vi "DETH_GPIT_COMBI_VR_COM5_COM7_hex_VE_FP_STOP_VE_BR_NEW.vi"() -> ()   [LabVIEW 2009]
uses:
  <vilib>/Instr/_visa.llb/VISA Configure Serial Port (Instr).vi
panel:
  in  "GPIT Backlash":i32
  in  "DETT Backlash":i32
  in  "DETH/GPIT":dbl max=1.0 step=1.0
  out "GPIT Status":string
  out "read buffer 3":string
  out "GPIT":i32
  out "GPIT Range?":bool
  out "GPIT rev/sec":dbl caption="Velocity"
  out "GPIT MINPOS":i32=-94296
  out "GPIT MAXPOS":i32=-34296
  out "GPIT COM PORT":refnum<visa-resource-name>="COM5"
  out "GPIT Step":i32
  in  "Stop":bool
  out "DETH Range?":bool
  out "DETH":i32
  out "read buffer 2":string
  out "DETH Status":string
  out "DETH rev//sec":dbl caption="Velocity"
  in  "Go":bool
  in  "DETH Step":i32=-1000 min=-1000 max=1000 step=100
  out "DETH MINPOS":i32=-94296
  out "DETH MAXPOS":i32=-34296
  out "DETT COM PORT":refnum<visa-resource-name>="COM5"
  # "DETH COM5 & GPIT COM7"
  # "20000 steps/rev\n2.5mm/rev\n0.05rev/sec"
  # "20000 steps/rev\n1 mm/rev\n0.01rev/sec"
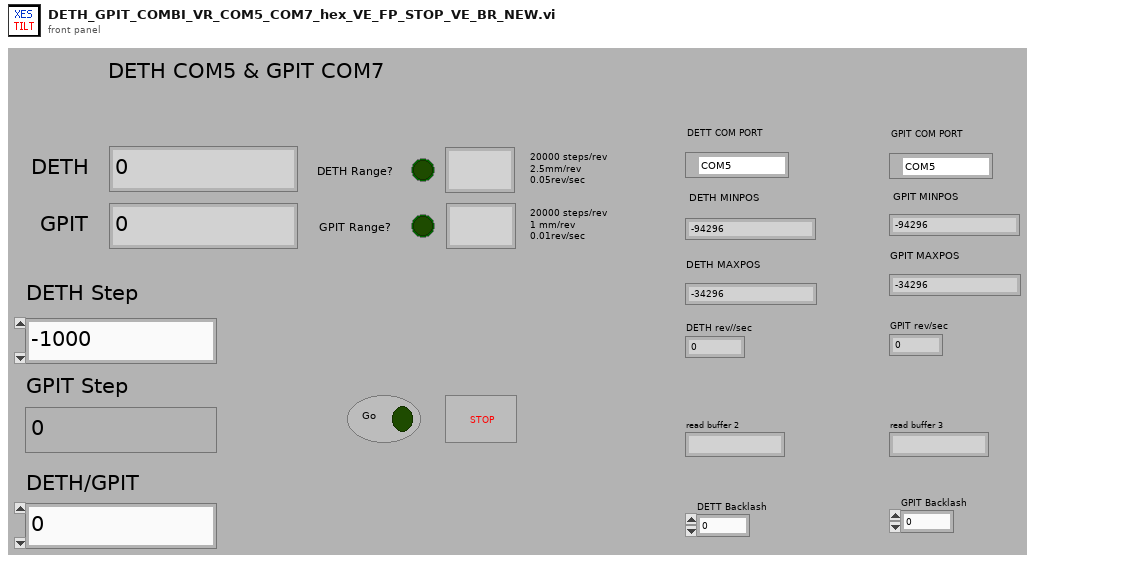
[diagram p1: front panel]
types:
  T1 = enum16{"Power-up Signature", "Accel Rate", "Accel Max", "Bit Rate", "Buffer Status", "Change Current", "Commence Jogging", "Change Jog Speed", "Continue", "Define Address", "Distance for FC,FM,FO,FY", "Decel Rate", "Distance or Position", "Define Limits", "Encoder Deadband", "Encoder Function", "Encoder Position", "Encoder Ratio", "Feed to Length with Speed Change", "Feed to Length", "Feed to Sensor with Mask Dist", "Feed to Length & Set Output", "Feed to Position", "Feed to Sensor", "Feed to Sensor w/safety", "Follow Handwheel", "Immediate Distance?", "Immediate Encoder?", "Immediate Low Output", "Immediate High Output", "Immediate Position?", "Input Status?", "Jog Accel/Decel", "Jog Disable", "Jog Enable", "Jog Speed", "Motor Disable", "Motor Enable", "Microstep Resolution", "Power up Current", "Power up Mode", "Pause", "Request Status", "Revision Level?", "Seek Home", "Stop Jogging", "Stop & Kill Buffer", "Set Output", "Set ABS Position", "Send String", "Stop", "Velocity for Speed Change", "Velocity Setting", "Wait for Input", "Wait Time"}
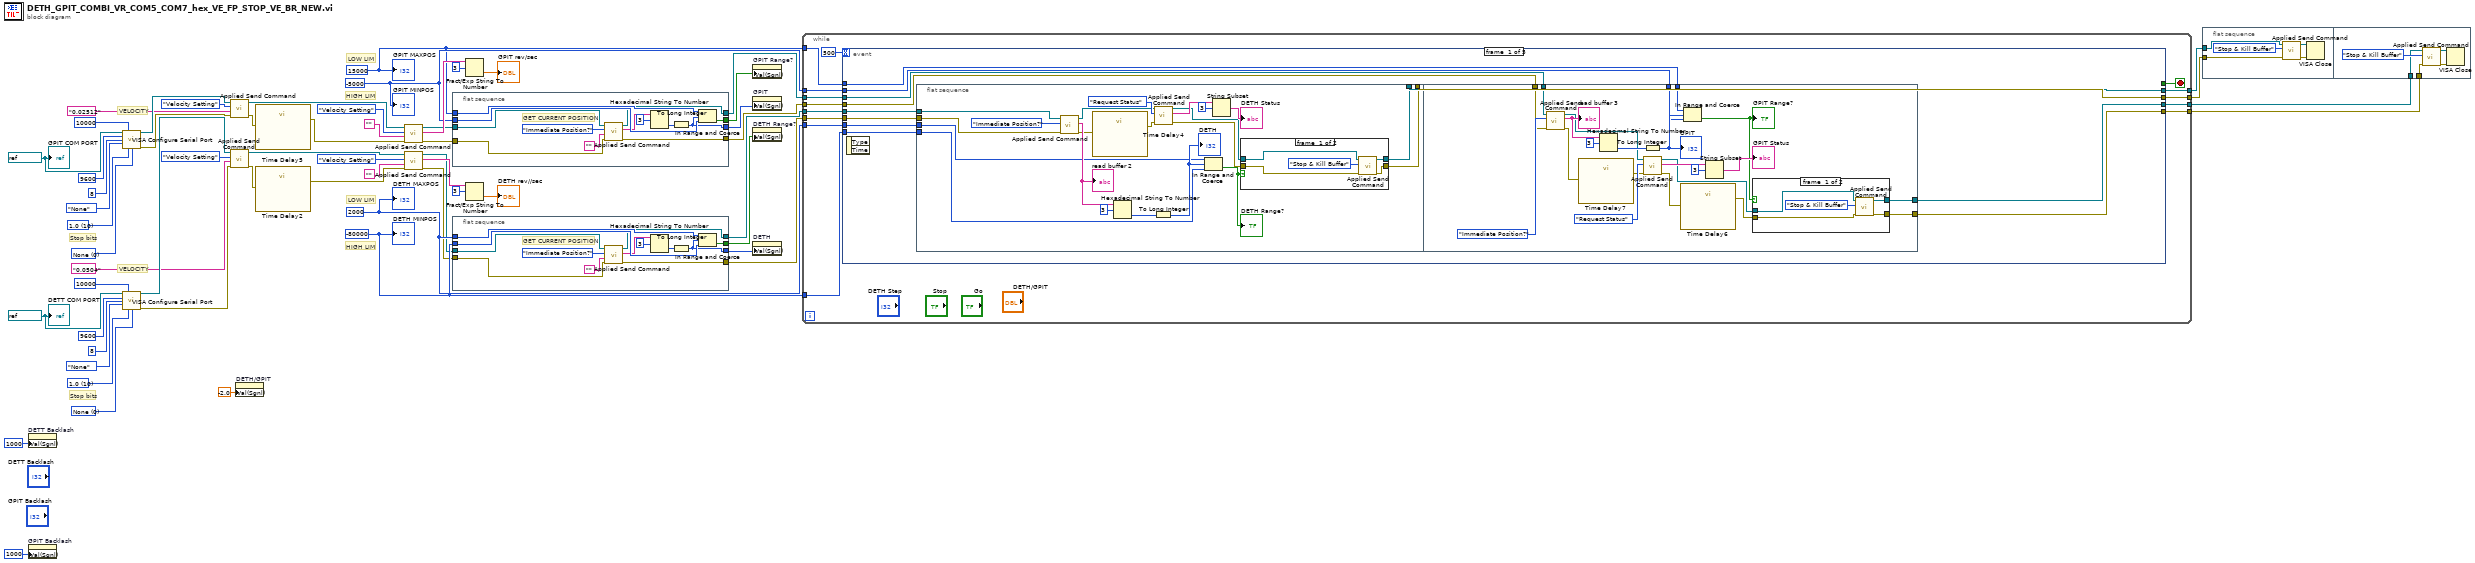
[diagram p0: block diagram]
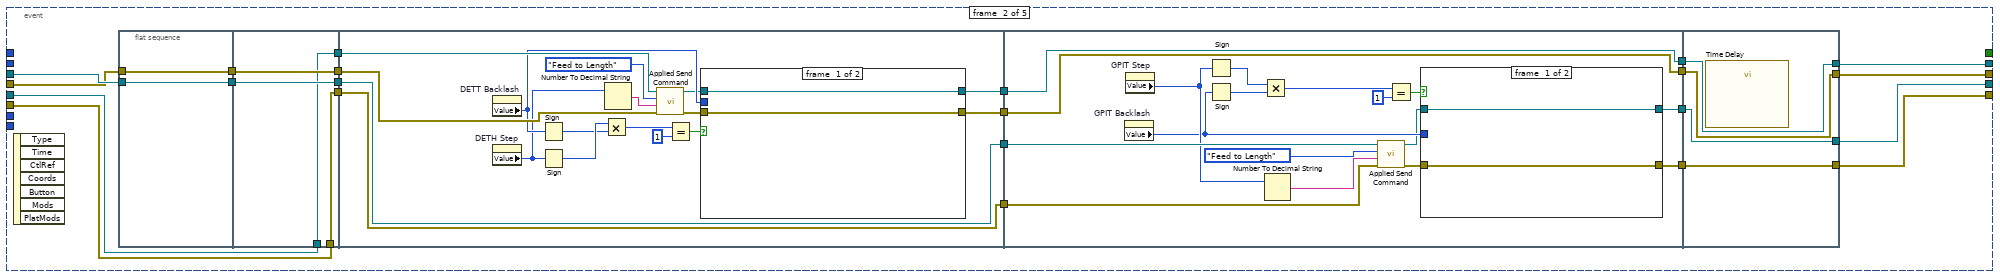
[diagram p4: hidden frame]
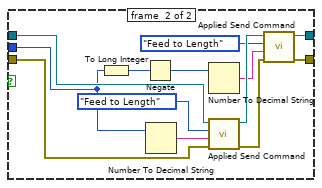
[diagram p5: hidden frame]
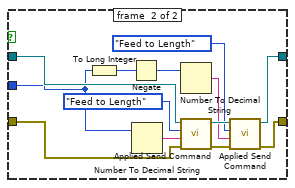
[diagram p6: hidden frame]
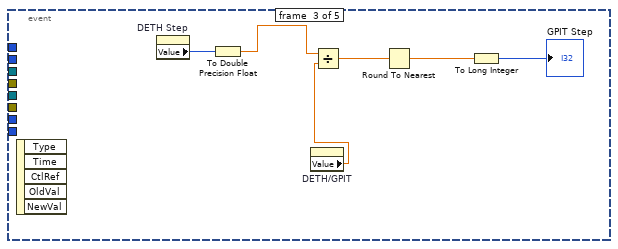
[diagram p7: hidden frame]
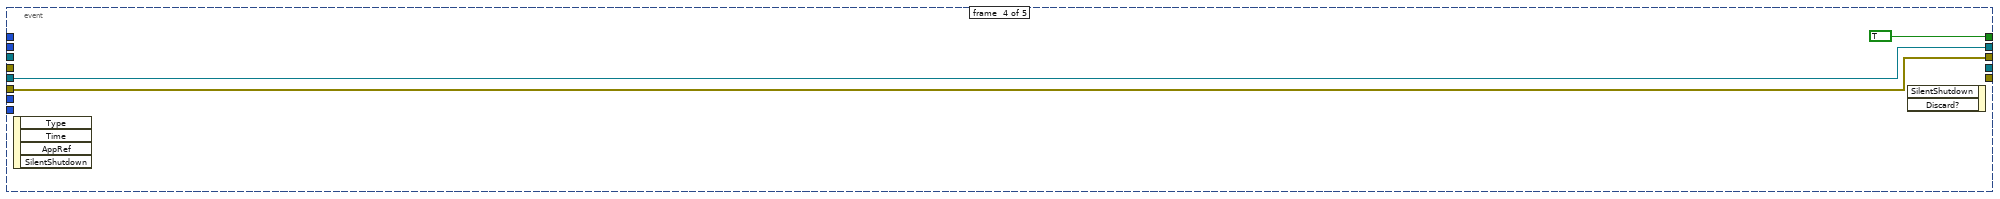
[diagram p8: hidden frame]
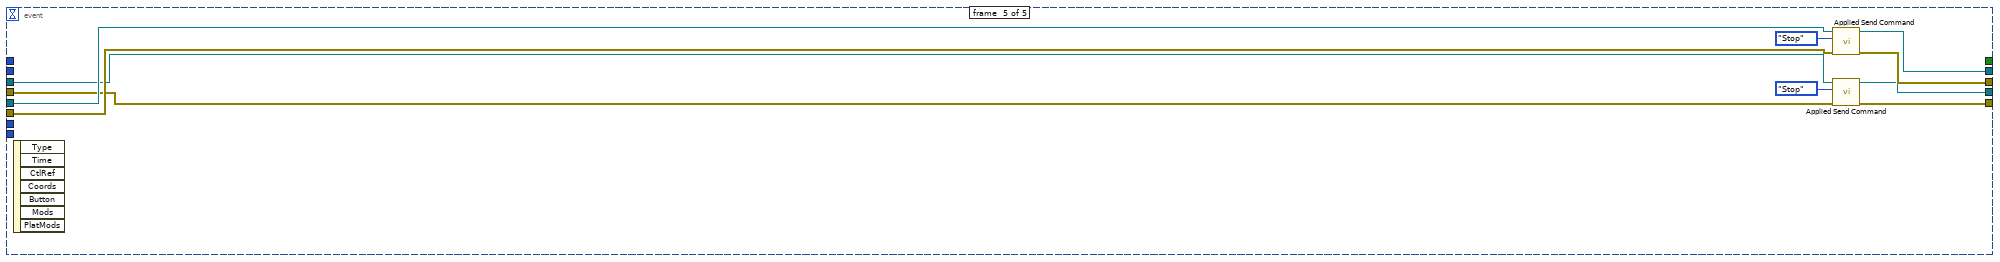
[diagram p9: hidden frame]
diagram:
  w12 = -5000 ("lower limit")
  w11 = 15000 ("upper limit")
  w27 = refnum<visa-resource-name> "COM7" ("COM PORT")
  w29 = u16 0 items=["None", "XON/XOFF", "RTS/CTS", "XON/XOFF & RTS/CTS", "DTR/DSR", "XON/XOFF & DTR/DSR"] ("flow control (0:none)")
  w30 = u16 10 items=["1.0"=10, "1.5"=15, "2.0"=20] ("stop bits (10: 1 bit)")
  w51 = -80000 ("lower limit")
  w52 = 2000 ("upper limit")
  w55 = refnum<visa-resource-name> "COM5" ("COM PORT")
  w57 = u16 0 items=["None", "XON/XOFF", "RTS/CTS", "XON/XOFF & RTS/CTS", "DTR/DSR", "XON/XOFF & DTR/DSR"] ("flow control (0:none)")
  w58 = u16 10 items=["1.0"=10, "1.5"=15, "2.0"=20] ("stop bits (10: 1 bit)")
  # "VELOCITY"
  # "HIGH LIM"
  # "LOW LIM"
  # "Stop bits"
  # "VELOCITY"
  # "HIGH LIM"
  # "LOW LIM"
  # "Stop bits"
  n1 = property on="DETT Backlash" class="DigNum (strict)"("Val(Sgnl)"=1000 ("Value (Signaling)")) -> ()  [unwired: 2 in, 2 out]
  n2 = property on="GPIT Backlash" class="DigNum (strict)"("Val(Sgnl)"=1000 ("Value (Signaling)")) -> ()  [unwired: 2 in, 2 out]
  n3 = call-poly "VISA Configure Serial Port"("VISA resource name"=w27, "timeout (10sec)"=u32 10000, "baud rate (9600)"=u32 9600, "data bits (8)"=u16 8, "parity (0:none)"=enum16{"None", "Odd", "Even", "Mark", "Space"}."None", "stop bits (10: 1 bit)"=w30, "flow control (0:none)"=w29) -> ("VISA resource name out"=w15:refnum<visa-resource-name>, "error out"=w14:errorcluster)  [unwired: 7 in]
  n4 = call-poly "VISA Configure Serial Port"("VISA resource name"=w55, "timeout (10sec)"=u32 10000, "baud rate (9600)"=u32 9600, "data bits (8)"=u16 8, "parity (0:none)"=enum16{"None", "Odd", "Even", "Mark", "Space"}."None", "stop bits (10: 1 bit)"=w58, "flow control (0:none)"=w57) -> ("VISA resource name out"=w37:refnum<visa-resource-name>, "error out"=w36:errorcluster)  [unwired: 7 in]
  n5 = call "Applied Send Command.vi"("error in (no error)"=w14, "Extra"="0.02512", "Command"=T1."Velocity Setting", "VISA resource name"=w15) -> ("error out"=w25:errorcluster, "VISA resource name out"=w20:refnum<visa-resource-name>)  [unwired: 3 in, 1 out]
  n6 = call "Applied Send Command.vi"("error in (no error)"=w36, "Extra"="0.0504", "Command"=T1."Velocity Setting", "VISA resource name"=w37) -> ("error out"=w49:errorcluster, "VISA resource name out"=w44:refnum<visa-resource-name>)  [unwired: 3 in, 1 out]
  n7 = property on="DETH/GPIT" class="DigNum (strict)"("Val(Sgnl)"=-2.0 ("Value (Signaling)")) -> ()  [unwired: 2 in, 2 out]
  n8 = call "Time Delay5"("error in (no error)"=w25) -> ("error out"=w21:errorcluster)  [unwired: 10 in]
  n9 = call "Time Delay2"("error in (no error)"=w49) -> ("error out"=w45:errorcluster)  [unwired: 10 in]
  n10 = call "Applied Send Command.vi"("error in (no error)"=w21, "Extra"="", "Command"=T1."Velocity Setting", "VISA resource name"=w20) -> ("error out"=w18:errorcluster, "read buffer"=w23:string, "VISA resource name out"=w19:refnum<visa-resource-name>)  [unwired: 3 in]
  n11 = call "Applied Send Command.vi"("error in (no error)"=w45, "Extra"="", "Command"=T1."Velocity Setting", "VISA resource name"=w44) -> ("error out"=w42:errorcluster, "read buffer"=w47:string, "VISA resource name out"=w43:refnum<visa-resource-name>)  [unwired: 3 in]
  n12 = flat-sequence {
    tunnel: w18 -> [w74]
    tunnel: w19 -> [w73]
    tunnel: w11 -> [w71]
    tunnel: w12 -> [w70]
    tunnel: [w72] -> w9
    tunnel: [w62] -> w4
    tunnel: [w69] -> w6
    tunnel: [w68] -> w10
    frame #0 {
      # "GET CURRENT POSITION"
      n13 = call "Applied Send Command.vi"("error in (no error)"=w74, "Extra"="", "Command"=T1."Immediate Position?", "VISA resource name"=w73) -> ("error out"=w72:errorcluster, "read buffer"=w66:string, "VISA resource name out"=w68:refnum<visa-resource-name>)  [unwired: 3 in]
      n14 = Hexadecimal String To Number(string=w66, offset=3) -> (number=w63:u32)  [unwired: 1 in, 1 out]
      n15 = To Long Integer(number=w63) -> (32bit integer=w62:i32)
      n16 = In Range and Coerce(upper limit=w71, x=w62, lower limit=w70) -> (In Range?=w69:bool)  [unwired: 1 out]
    }
  }
  n17 = flat-sequence {
    tunnel: w42 -> [w87]
    tunnel: w43 -> [w86]
    tunnel: w52 -> [w85]
    tunnel: w51 -> [w84]
    tunnel: [w75] -> w53
    tunnel: [w76] -> w5
    tunnel: [w83] -> w34
    tunnel: [w82] -> w54
    frame #0 {
      # "GET CURRENT POSITION"
      n18 = call "Applied Send Command.vi"("error in (no error)"=w87, "Extra"="", "Command"=T1."Immediate Position?", "VISA resource name"=w86) -> ("error out"=w75:errorcluster, "read buffer"=w80:string, "VISA resource name out"=w82:refnum<visa-resource-name>)  [unwired: 3 in]
      n19 = Hexadecimal String To Number(string=w80, offset=3) -> (number=w77:u32)  [unwired: 1 in, 1 out]
      n20 = To Long Integer(number=w77) -> (32bit integer=w76:i32)
      n21 = In Range and Coerce(upper limit=w85, x=w76, lower limit=w84) -> (In Range?=w83:bool)  [unwired: 1 out]
    }
  }
  n22 = Fract/Exp String To Number(string=w23, offset=3) -> (number=→"GPIT rev/sec":dbl)  [unwired: 2 in, 1 out]
  n23 = Fract/Exp String To Number(string=w47, offset=3) -> (number=→"DETH rev//sec":dbl)  [unwired: 2 in, 1 out]
  n24 = property on="GPIT Range?" class="Bool (strict)"("Val(Sgnl)"=w6) -> ()  [unwired: 2 in, 2 out]
  n25 = property on="GPIT" class="DigNum (strict)"("Val(Sgnl)"=w4) -> ()  [unwired: 2 in, 2 out]
  n26 = property on="DETH Range?" class="Bool (strict)"("Val(Sgnl)"=w34) -> ()  [unwired: 2 in, 2 out]
  n27 = property on="DETH" class="DigNum (strict)"("Val(Sgnl)"=w5) -> ()  [unwired: 2 in, 2 out]
  n28 = while {
    tunnel: w54 -> [w95]
    tunnel: w53 -> [w100]
    tunnel: [w101] -> w38
    tunnel: [w99] -> w39
    tunnel: w52 -> [w98]
    tunnel: w51 -> [w97]
    tunnel: w12 -> [w93]
    tunnel: w11 -> [w88]
    tunnel: w10 -> [w92]
    tunnel: w9 -> [w91]
    tunnel: [w90] -> w8
    tunnel: [w89] -> w7
    stop <- w94 stop-if-true
    n29 = event shown="[1] \"Go\": Mouse Up" {
      selector: _ -> [_ _ _ _ _]
      dyn-events: _ -> [_ _ _ _ _]
      timeout: 500 -> [_ _ _ _ _]
      tunnel: w100 -> [w111 w172 _ w274 w283]
      tunnel: [w105 w179 _ w274 w281] -> w101
      tunnel: w95 -> [w110 w171 _ w275 w284]
      tunnel: [w104 w192 _ w275 w282] -> w99
      tunnel: w98 -> [w113 _ _ _ _]
      tunnel: w97 -> [w112 _ _ _ _]
      tunnel: [_ _ _ TRUE _] -> w94
      tunnel: w93 -> [w102 _ _ _ _]
      tunnel: w88 -> [w103 _ _ _ _]
      tunnel: w92 -> [w109 w187 _ _ w277]
      tunnel: w91 -> [w108 w183 _ _ w276]
      tunnel: [w107 w177 _ _ w279] -> w90
      tunnel: [w106 w175 _ _ w278] -> w89
      event #0 {
        n30 = event-data() -> ()  [unwired: 1 in, 2 out]
        n31 = flat-sequence {
          tunnel: w112 -> [w134]
          tunnel: w113 -> [w126]
          tunnel: w111 -> [w125]
          tunnel: w110 -> [w124]
          tunnel: [w116] -> w104
          tunnel: [w114] -> w105
          tunnel: w109 -> [w150]
          tunnel: w108 -> [w149]
          tunnel: w103 -> [w148]
          tunnel: w102 -> [w147]
          tunnel: [w144] -> w107
          tunnel: [w145] -> w106
          frame #0 {
            n32 = call "Applied Send Command.vi"("error in (no error)"=w125, "Command"=T1."Immediate Position?", "VISA resource name"=w124) -> ("error out"=w120:errorcluster, "read buffer"=w132:string, "VISA resource name out"=w127:refnum<visa-resource-name>)  [unwired: 4 in]
            "read buffer 2" <- w132
            n33 = call "Time Delay4"("error in (no error)"=w120) -> ("error out"=w119:errorcluster)  [unwired: 10 in]
            n34 = Hexadecimal String To Number(string=w132, offset=3) -> (number=w131:u32)  [unwired: 1 in, 1 out]
            n35 = call "Applied Send Command.vi"("error in (no error)"=w119, "Command"=T1."Request Status", "VISA resource name"=w127) -> ("error out"=w115:errorcluster, "read buffer"=w123:string, "VISA resource name out"=w117:refnum<visa-resource-name>)  [unwired: 4 in]
            n36 = To Long Integer(number=w131) -> (32bit integer=w129:i32)
            "DETH" <- w129
            n37 = In Range and Coerce(upper limit=w126, x=w129, lower limit=w134) -> (In Range?=w118:bool)  [unwired: 1 out]
            "DETH Range?" <- w118
            n38 = String Subset(string=w123, offset (0)=3) -> (substring=→"DETH Status":string)  [unwired: 1 in]
            n39 = case shown="False" w118 {
              tunnel: w117 -> [w136 w141]
              tunnel: [w138 w141] -> w116
              tunnel: [w139 w140] -> w114
              tunnel: w115 -> [w135 w140]
              frame #0 {
                n40 = call "Applied Send Command.vi"("error in (no error)"=w135, "Command"=T1."Stop & Kill Buffer", "VISA resource name"=w136) -> ("error out"=w139:errorcluster, "VISA resource name out"=w138:refnum<visa-resource-name>)  [unwired: 4 in, 1 out]
              }
              frame #1 {
              }
            }
          }
          frame #1 {
            n41 = call "Applied Send Command.vi"("error in (no error)"=w149, "Command"=T1."Immediate Position?", "VISA resource name"=w150) -> ("error out"=w152:errorcluster, "read buffer"=w162:string, "VISA resource name out"=w157:refnum<visa-resource-name>)  [unwired: 4 in]
            "read buffer 3" <- w162
            n42 = call "Time Delay7"("error in (no error)"=w152) -> ("error out"=w151:errorcluster)  [unwired: 10 in]
            n43 = Hexadecimal String To Number(string=w162, offset=3) -> (number=w161:u32)  [unwired: 1 in, 1 out]
            n44 = To Long Integer(number=w161) -> (32bit integer=w159:i32)
            "GPIT" <- w159
            n45 = call "Applied Send Command.vi"("error in (no error)"=w151, "Command"=T1."Request Status", "VISA resource name"=w157) -> ("error out"=w156:errorcluster, "read buffer"=w155:string, "VISA resource name out"=w143:refnum<visa-resource-name>)  [unwired: 4 in]
            n46 = call "Time Delay6"("error in (no error)"=w156) -> ("error out"=w146:errorcluster)  [unwired: 10 in]
            n47 = In Range and Coerce(upper limit=w148, x=w159, lower limit=w147) -> (In Range?=w142:bool)  [unwired: 1 out]
            "GPIT Range?" <- w142
            n48 = String Subset(string=w155, offset (0)=3) -> (substring=→"GPIT Status":string)  [unwired: 1 in]
            n49 = case shown="False" w142 {
              tunnel: w143 -> [w165 w170]
              tunnel: [w167 w170] -> w144
              tunnel: [w168 w169] -> w145
              tunnel: w146 -> [w164 w169]
              frame #0 {
                n50 = call "Applied Send Command.vi"("error in (no error)"=w164, "Command"=T1."Stop & Kill Buffer", "VISA resource name"=w165) -> ("error out"=w168:errorcluster, "VISA resource name out"=w167:refnum<visa-resource-name>)  [unwired: 4 in, 1 out]
              }
              frame #1 {
              }
            }
          }
        }
      }
      event #1 {
        n51 = event-data() -> ()  [unwired: 1 in, 7 out]
        n52 = flat-sequence {
          tunnel: w187 -> [w194]
          tunnel: [w194] -> w186
          tunnel: [w193] -> w184
          tunnel: w183 -> [w193]
          tunnel: [w198] -> w189
          tunnel: w186 -> [w198]
          tunnel: [w197] -> w185
          tunnel: w184 -> [w197]
          tunnel: [w196] -> w174
          tunnel: [w195] -> w173
          tunnel: w172 -> [w195]
          tunnel: w171 -> [w196]
          tunnel: [w200] -> w191
          tunnel: w189 -> [w214]
          tunnel: [w214] -> w188
          tunnel: w185 -> [w212]
          tunnel: [w211] -> w182
          tunnel: [w199] -> w181
          tunnel: w174 -> [w213]
          tunnel: w173 -> [w211]
          tunnel: w191 -> [w247]
          tunnel: [w247] -> w190
          tunnel: w188 -> [w245]
          tunnel: w182 -> [w244]
          tunnel: w181 -> [w243]
          tunnel: [w243] -> w180
          tunnel: [w231] -> w178
          tunnel: [w233] -> w176
          tunnel: [w266] -> w192
          tunnel: w190 -> [w266]
          tunnel: w180 -> [w265]
          tunnel: [w265] -> w179
          tunnel: w178 -> [w264]
          tunnel: [w264] -> w177
          tunnel: [w263] -> w175
          tunnel: w176 -> [w263]
          frame #0 {
          }
          frame #1 {
          }
          frame #2 {
            n53 = property on="DETT Backlash" class="DigNum (strict)"() -> ("Value"=w204:i32)  [unwired: 2 in, 2 out]
            n54 = property on="DETH Step" class="DigNum (strict)"() -> ("Value"=w203:i32)  [unwired: 2 in, 2 out]
            n55 = Sign(1:w204) -> (0:w208:i32)
            n56 = Sign(1:w203) -> (0:w209:i32)
            n57 = Multiply(x=w209, y=w208) -> (x*y=w207:i32)
            n58 = Number To Decimal String(number=w203) -> (decimal integer string=w210:string)  [unwired: 1 in]
            n59 = call "Applied Send Command.vi"("error in (no error)"=w212, "Extra"=w210, "Command"=T1."Feed to Length", "VISA resource name"=w213) -> ("error out"=w201:errorcluster, "VISA resource name out"=w202:refnum<visa-resource-name>)  [unwired: 3 in, 1 out]
            n60 = Equal?(x=w207, y=1) -> (x = y?=w205:bool)
            n61 = case shown="True" w205 {
              tunnel: w202 -> [w217 w229]
              tunnel: [w217 w223] -> w200
              tunnel: [w216 w224] -> w199
              tunnel: w201 -> [w216 w228]
              tunnel: w204 -> [_ w218]
              frame #0 {
              }
              frame #1 {
                n62 = To Long Integer(number=w218) -> (32bit integer=w221:i32)
                n63 = Negate(x=w221) -> (-x=w222:i32)
                n64 = Number To Decimal String(number=w218) -> (decimal integer string=w227:string)  [unwired: 1 in]
                n65 = Number To Decimal String(number=w222) -> (decimal integer string=w220:string)  [unwired: 1 in]
                n66 = call "Applied Send Command.vi"("error in (no error)"=w228, "Extra"=w227, "Command"=T1."Feed to Length", "VISA resource name"=w229) -> ("error out"=w225:errorcluster, "VISA resource name out"=w226:refnum<visa-resource-name>)  [unwired: 3 in, 1 out]
                n67 = call "Applied Send Command.vi"("error in (no error)"=w225, "Extra"=w220, "Command"=T1."Feed to Length", "VISA resource name"=w226) -> ("error out"=w224:errorcluster, "VISA resource name out"=w223:refnum<visa-resource-name>)  [unwired: 3 in, 1 out]
              }
            }
          }
          frame #3 {
            n68 = property on="GPIT Backlash" class="DigNum (strict)"() -> ("Value"=w235:i32)  [unwired: 2 in, 2 out]
            n69 = property on="GPIT Step" class="DigNum (strict)"() -> ("Value"=w237:i32)  [unwired: 2 in, 2 out]
            n70 = Sign(1:w237) -> (0:w241:i32)
            n71 = Sign(1:w235) -> (0:w240:i32)
            n72 = Multiply(x=w241, y=w240) -> (x*y=w239:i32)
            n73 = Number To Decimal String(number=w237) -> (decimal integer string=w242:string)  [unwired: 1 in]
            n74 = call "Applied Send Command.vi"("error in (no error)"=w244, "Extra"=w242, "Command"=T1."Feed to Length", "VISA resource name"=w245) -> ("error out"=w234:errorcluster, "VISA resource name out"=w232:refnum<visa-resource-name>)  [unwired: 3 in, 1 out]
            n75 = Equal?(x=w239, y=1) -> (x = y?=w236:bool)
            n76 = case shown="True" w236 {
              tunnel: w232 -> [w249 w261]
              tunnel: [w249 w255] -> w231
              tunnel: [w248 w256] -> w233
              tunnel: w234 -> [w248 w260]
              tunnel: w235 -> [_ w250]
              frame #0 {
              }
              frame #1 {
                n77 = To Long Integer(number=w250) -> (32bit integer=w253:i32)
                n78 = Negate(x=w253) -> (-x=w254:i32)
                n79 = Number To Decimal String(number=w250) -> (decimal integer string=w259:string)  [unwired: 1 in]
                n80 = Number To Decimal String(number=w254) -> (decimal integer string=w252:string)  [unwired: 1 in]
                n81 = call "Applied Send Command.vi"("error in (no error)"=w260, "Extra"=w259, "Command"=T1."Feed to Length", "VISA resource name"=w261) -> ("error out"=w257:errorcluster, "VISA resource name out"=w258:refnum<visa-resource-name>)  [unwired: 3 in, 1 out]
                n82 = call "Applied Send Command.vi"("error in (no error)"=w257, "Extra"=w252, "Command"=T1."Feed to Length", "VISA resource name"=w258) -> ("error out"=w256:errorcluster, "VISA resource name out"=w255:refnum<visa-resource-name>)  [unwired: 3 in, 1 out]
              }
            }
          }
          frame #4 {
            n83 = call "Time Delay"() -> ()  [unwired: 11 in, 1 out]
          }
        }
      }
      event #2 {
        n84 = event-data() -> ()  [unwired: 1 in, 5 out]
        n85 = property on="DETH Step" class="DigNum (strict)"() -> ("Value"=w268:i32)  [unwired: 2 in, 2 out]
        n86 = To Double Precision Float(number=w268) -> (double precision float=w269:dbl)
        n87 = property on="DETH/GPIT" class="DigNum (strict)"() -> ("Value"=w267:dbl)  [unwired: 2 in, 2 out]
        n88 = Divide(x=w269, y=w267) -> (x/y=w272:dbl)
        n89 = Round To Nearest(number=w272) -> (nearest integer value=w271:dbl)
        n90 = To Long Integer(number=w271) -> (32bit integer=→"GPIT Step":i32)
      }
      event #3 {
        n91 = event-data() -> ()  [unwired: 1 in, 4 out]
        n92 = event-data() -> ()  [unwired: 3 in, 1 out]
      }
      event #4 {
        n93 = event-data() -> ()  [unwired: 1 in, 7 out]
        n94 = call "Applied Send Command.vi"("error in (no error)"=w283, "Command"=T1."Stop", "VISA resource name"=w284) -> ("error out"=w281:errorcluster, "VISA resource name out"=w282:refnum<visa-resource-name>)  [unwired: 4 in, 1 out]
        n95 = call "Applied Send Command.vi"("error in (no error)"=w276, "Command"=T1."Stop", "VISA resource name"=w277) -> ("error out"=w278:errorcluster, "VISA resource name out"=w279:refnum<visa-resource-name>)  [unwired: 4 in, 1 out]
      }
    }
  }
  n96 = flat-sequence {
    tunnel: w39 -> [w289]
    tunnel: w38 -> [w286]
    tunnel: w8 -> [w291]
    tunnel: w7 -> [w292]
    frame #0 {
      n97 = call "Applied Send Command.vi"("error in (no error)"=w286, "Command"=T1."Stop & Kill Buffer", "VISA resource name"=w289) -> ("error out"=w287:errorcluster, "VISA resource name out"=w288:refnum<visa-resource-name>)  [unwired: 4 in, 1 out]
      n98 = VISA Close(VISA resource name=w288, error in (no error)=w287) -> ()  [unwired: 1 out]
    }
    frame #1 {
      n99 = call "Applied Send Command.vi"("error in (no error)"=w292, "Command"=T1."Stop & Kill Buffer", "VISA resource name"=w291) -> ("error out"=w293:errorcluster, "VISA resource name out"=w294:refnum<visa-resource-name>)  [unwired: 4 in, 1 out]
      n100 = VISA Close(VISA resource name=w294, error in (no error)=w293) -> ()  [unwired: 1 out]
    }
  }
  "DETT COM PORT" <- w55
  "DETH MAXPOS" <- w52
  "DETH MINPOS" <- w51
  "GPIT COM PORT" <- w27
  "GPIT MAXPOS" <- w11
  "GPIT MINPOS" <- w12
